vi "Draw Polygon.vi"(8 "error in (no error)":errorcluster) -> (0 "error out":errorcluster)   [LabVIEW 2014]
uses:
  System.Drawing
  C:/Robotic Systems/Products/AgFalcon/Software/Ground Station/Data/Mapping DLL/GMap.NET.WindowsForms.dll
  Data/Mapping DLL/GMap.NET.WindowsForms.dll
  Reference/SubVI/Main Map Control Refernce.vi
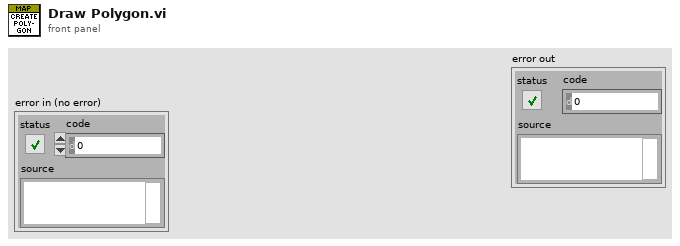
[diagram p1: front panel]
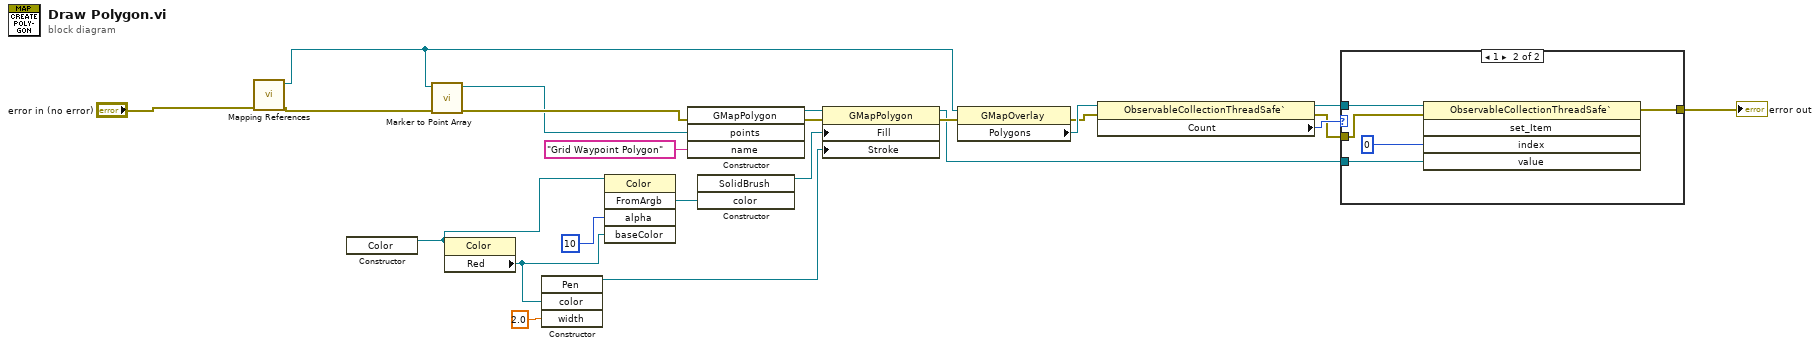
[diagram p0: block diagram]
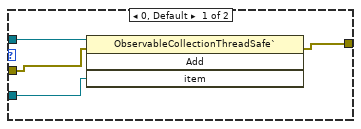
[diagram p2: hidden frame]
diagram:
  n1 = call-poly "Mapping References.vi"("Error In"="error in (no error)") -> ("Error Out"=w3:errorcluster, "Main Map Reference"=w1:refnum<k24>)  [unwired: 9 in]
  n2 = constructor class="Color"() -> (reference out=w15:refnum<k24>)  [unwired: 3 in, 2 out]
  n3 = call "Marker to Point Array.vi"("error in (no error)"=w3, "Overlay Ref"=w1) -> ("error out"=w12:errorcluster, "Point Array"=w11:refnum<k24>)  [unwired: 8 in]
  n4 = property class="Color"(reference=w15) -> ("Red"=w18:refnum<k24>)  [unwired: 1 in, 2 out]
  n5 = constructor class="Pen"("color"=w18, "width"=sgl 2.0 ("Width")) -> (reference out=w17:refnum<k24>)  [unwired: 3 in, 4 out]
  n6 = invoke class="Color" method="FromArgb"(reference=w15, "alpha"=10, "baseColor"=w18) -> ("FromArgb"=w16:refnum<k24>)  [unwired: 2 in, 4 out]
  n7 = constructor class="GMapPolygon"(error in=w12, "points"=w11, "name"="Grid Waypoint Polygon") -> (reference out=w22:refnum<k24>, error out=w21:errorcluster)  [unwired: 2 in, 3 out]
  n8 = constructor class="SolidBrush"("color"=w16) -> (reference out=w20:refnum<k24>)  [unwired: 3 in, 3 out]
  n9 = property class="GMapPolygon"(reference=w22, error in=w21, "Fill"=w20, "Stroke"=w17) -> (reference out=w10:refnum<k24>, error out=w14:errorcluster)
  n10 = property class="GMapOverlay"(reference=w1, error in=w14) -> (error out=w8:errorcluster, "Polygons"=w9:refnum<k24>)  [unwired: 1 out]
  n11 = property class="ObservableCollectionThreadSafe`"(reference=w9, error in=w8) -> (reference out=w5:refnum<k24>, error out=w4:errorcluster, "Count"=w6:i32)
  n12 = case shown="1" w6 {
    tunnel: w10 -> [w24 w32]
    tunnel: w5 -> [w26 w30]
    tunnel: [w25 w29] -> w7
    tunnel: w4 -> [w27 w28]
    frame 0, Default {
      n13 = invoke class="ObservableCollectionThreadSafe`" method="Add"(reference=w26, error in=w27, "item"=w24) -> (error out=w25:errorcluster)  [unwired: 1 in, 3 out]
    }
    frame 1 {
      n14 = invoke class="ObservableCollectionThreadSafe`" method="set_Item"(reference=w30, error in=w28, "index"=0, "value"=w32) -> (error out=w29:errorcluster)  [unwired: 1 in, 4 out]
    }
  }
  "error out" <- w7
